vi "ArrayToTuple.vi"(11 "Tableau":string[](array[string])) -> (3 "Tuple":string)   [LabVIEW 2020]
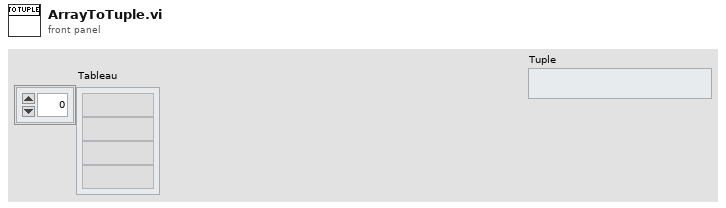
[diagram p1: front panel]
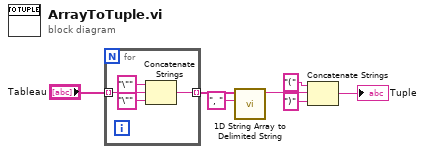
[diagram p0: block diagram]
diagram:
  n1 = for {
    tunnel: "Tableau" -> [w11] mode=indexing
    tunnel: [w8] -> w1 mode=indexing
    n2 = Concatenate Strings("\"" ("chaîne"), w11, "\"" ("chaîne")) -> (w8:string)
  }
  n3 = call <vilib>:"1D String Array to Delimited String.vi"("delimiter"=", ", "string array"=w1) -> ("delimited string"=w6:string)  [unwired: 9 in]
  n4 = Concatenate Strings("(", w6, ")" ("chaîne")) -> (→"Tuple":string)
